vi "Set Fullscale Accel Range.vi"(7 "I2C Channel":u8, 8 "Error In":errorcluster, 9 "Accel Full Scale Range":T1, 10 "Device Address":T8=enum."0x69", 11 "LINX Resource":T2) -> (0 "Error Out":errorcluster, 3 "LINX Resource":T2)   [LabVIEW 2020, in "LMH-LINX.lvlib" / "MPU60X0.lvlib"]
uses:
  MPU60X0.lvlib
  DeviceAddresses.ctl
  Private/Type Defs/LINX Ref.ctl
  Private/Type Defs/Platform.ctl
  Private/Type Defs/Interface.ctl
  Private/Device/Type Defs/LINX Device Config.ctl
  Private/Device/Type Defs/TCP Config.ctl
  Private/Device/Type Defs/Channels.ctl
  AccelFullScaleRanges.ctl
  RegisterAddresses.ctl
  Private/Local IO/LinxI2cWrite.vi
  Utilities/Check Channel.vi
  Private/Utilties/Generate Error.vi
  LMH-LINX.lvlib
  Private/Device/Device.lvlib
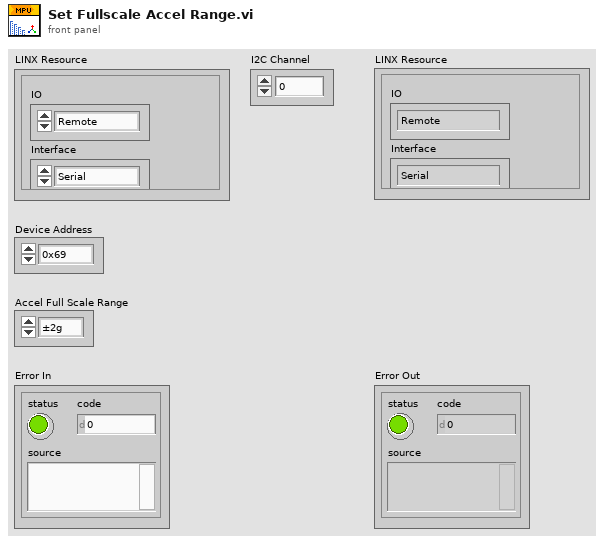
[diagram p1: front panel]
types:
  T1 = typedef "LMH-LINX.lvlib/MPU60X0.lvlib/AccelFullScaleRanges.ctl" = enum16{"±2g", "±4g", "±8g", "±16g"}
  T2 = typedef "LMH-LINX.lvlib/LINX Ref.ctl" = cluster{"IO":T3, "Interface":T4, "LINX Device Config":T5}
  T3 = typedef "LMH-LINX.lvlib/Platform.ctl" = enum16{"Remote", "Local"}
  T4 = typedef "LMH-LINX.lvlib/Interface.ctl" = enum16{"Serial", "TCP"}
  T5 = typedef "LMH-LINX.lvlib/Device.lvlib/LINX Device Config.ctl" = cluster{"Interface":T4, "COM Port":refnum<visa-resource-name>, "TCP Configuration":T6, "Device Family":u8, "Device ID":u8, "Device Name":string, "TCP Ref":refnum<k5>, "Channels":T7}
  T6 = typedef "LMH-LINX.lvlib/Device.lvlib/TCP Config.ctl" = cluster{"IP Address":string, "Port":u16}
  T7 = typedef "LMH-LINX.lvlib/Channels.ctl" = cluster{"DI":u8[], "DO":u8[], "AI":u8[], "AO":u8[], "PWM":u8[], "QE":u8[], "UART":u8[], "I2C 2":u8[], "SPI":u8[], "CAN":u8[], "Servo":u8[], "AI Ref (V)":dbl, "AI Resolution (Bits)":u8, "AO Ref (V)":dbl, "AO Resolution (Bits)":u8}
  T8 = typedef "LMH-LINX.lvlib/MPU60X0.lvlib/DeviceAddresses.ctl" = enum16{"0x68", "0x69"}
  T9 = typedef "LMH-LINX.lvlib/MPU60X0.lvlib/RegisterAddresses.ctl" = u16
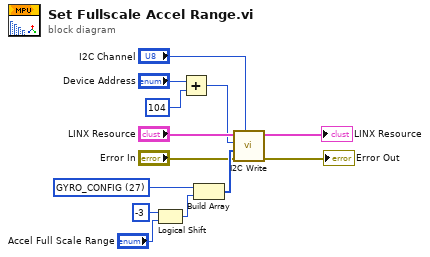
[diagram p0: block diagram]
diagram:
  w12 = T9 27 items=["SELF_TEST_X"=13, "SELF_TEST_Y"=14, "SELF_TEST_Z"=15, "SELF_TEST_A"=16, "SMPLRT_DIV"=25, "CONFIG"=26, "GYRO_CONFIG"=27, "ACCEL_CONFIG"=28, "MOT_THR"=31, "FIFO_EN"=35, "I2C_MST_CTRL"=36, "I2C_SLV0_ADDR"=37, "I2C_SLV0_REG"=38, "I2C_SLV0_CTRL"=39, "I2C_SLV1_ADDR"=40, "I2C_SLV1_REG"=41, "I2C_SLV1_CTRL"=42, "I2C_SLV2_ADDR"=43, "I2C_SLV2_REG"=44, "I2C_SLV2_CTRL"=45, "I2C_SLV3_ADDR"=46, "I2C_SLV3_REG"=47, "I2C_SLV3_CTRL"=48, "I2C_SLV4_ADDR"=49, "I2C_SLV4_REG"=50, "I2C_SLV4_DO"=51, "I2C_SLV4_CTRL"=52, "I2C_SLV4_DI"=53, "I2C_MST_STATUS"=54, "INT_PIN_CFG"=55, "INT_ENABLE"=56, "INT_STATUS"=58, "ACCEL_XOUT_H"=59, "ACCEL_XOUT_L"=60, "ACCEL_YOUT_H"=61, "ACCEL_YOUT_L"=62, "ACCEL_ZOUT_H"=63, "ACCEL_ZOUT_L"=64, "TEMP_OUT_H"=65, "TEMP_OUT_L"=66, "GYRO_XOUT_H"=67, "GYRO_XOUT_L"=68, "GYRO_YOUT_H"=69, "GYRO_YOUT_L"=70, "GYRO_ZOUT_H"=71, "GYRO_ZOUT_L"=72, "EXT_SENS_DATA_00"=73, "EXT_SENS_DATA_01"=74, "EXT_SENS_DATA_02"=75, "EXT_SENS_DATA_03"=76, "EXT_SENS_DATA_04"=77, "EXT_SENS_DATA_05"=78, "EXT_SENS_DATA_06"=79, "EXT_SENS_DATA_07"=80, "EXT_SENS_DATA_08"=81, "EXT_SENS_DATA_09"=82, "EXT_SENS_DATA_10"=83, "EXT_SENS_DATA_11"=84, "EXT_SENS_DATA_12"=85, "EXT_SENS_DATA_13"=86, "EXT_SENS_DATA_14"=87, "EXT_SENS_DATA_15"=88, "EXT_SENS_DATA_16"=89, "EXT_SENS_DATA_17"=90, "EXT_SENS_DATA_18"=91, "EXT_SENS_DATA_19"=92, "EXT_SENS_DATA_20"=93, "EXT_SENS_DATA_21"=94, "EXT_SENS_DATA_22"=95, "EXT_SENS_DATA_23"=96, "I2C_SLV0_DO"=99, "I2C_SLV1_DO"=100, "I2C_SLV2_DO"=101, "I2C_SLV3_DO"=102, "I2C_MST_DELAY_CTRL"=103, "SIGNAL_PATH_RESET"=104, "MOT_DETECT_CTRL"=105, "USER_CTRL"=106, "PWR_MGMT_1"=107, "PWR_MGMT_2"=108, "FIFO_COUNTH"=114, "FIFO_COUNTL"=115, "FIFO_R_W"=116, "WHO_AM_I"=117] ("Register Addresses")
  n1 = Logical Shift(y=i16 -3, x="Accel Full Scale Range") -> (x << y=w10:u32)
  n2 = Add(x="Device Address", y=104) -> (x+y=w1:i32)
  n3 = Build Array(w12, w10) -> (w13:u32[])
  n4 = call "I2C Write.vi"("I2C Channel"="I2C Channel", "Error In"="Error In", "Data"=w13, "I2C Slave Address (0)"=w1, "LINX Resource"="LINX Resource") -> ("Error Out"=→"Error Out":errorcluster, "LINX Resource"=→"LINX Resource":T2)  [unwired: 5 in]
